vi "4 Axis - Set Absolute Target Position.vi"(4 "error in (no error)":errorcluster, 5 "Positions":sgl[](array[numeric]), 7 "Controller Reference In":refnum<k7>) -> (0 "error out":errorcluster, 3 "Controller Reference Out":refnum<k7>)   [LabVIEW 2015]
doc: "Sets all 4 axis target positions (Absolute positions)."
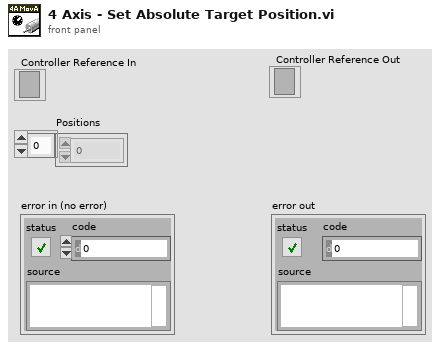
[diagram p1: front panel]
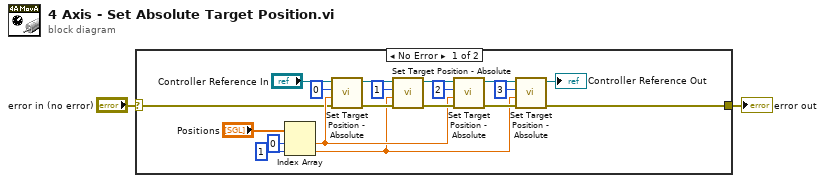
[diagram p0: block diagram]
diagram:
  n1 = case shown="No Error" "error in (no error)" {
    selector: "error in (no error)" -> [w3 w22]
    tunnel: [w4 w22] -> w2
    frame No Error {
      n2 = Index Array(array="Positions", index #1=0 ("index"), index #2=1 ("index")) -> (element #1=w8:sgl, element #2=w7:sgl)
      n3 = call "Set Target Position - Absolute.vi"("error in (no error)"=w3, "Target Position"=w8, "Axis In"=i16 0, "Controller Reference In"="Controller Reference In") -> ("error out"=w18:errorcluster, "Controller Reference Out"=w19:refnum<k7>)  [unwired: 1 in, 1 out]
      n4 = call "Set Target Position - Absolute.vi"("error in (no error)"=w18, "Target Position"=w7, "Axis In"=i16 1, "Controller Reference In"=w19) -> ("error out"=w16:errorcluster, "Controller Reference Out"=w17:refnum<k7>)  [unwired: 1 in, 1 out]
      n5 = call "Set Target Position - Absolute.vi"("error in (no error)"=w16, "Target Position"=w8, "Axis In"=i16 2, "Controller Reference In"=w17) -> ("error out"=w14:errorcluster, "Controller Reference Out"=w15:refnum<k7>)  [unwired: 1 in, 1 out]
      n6 = call "Set Target Position - Absolute.vi"("error in (no error)"=w14, "Target Position"=w7, "Axis In"=i16 3, "Controller Reference In"=w15) -> ("error out"=w4:errorcluster, "Controller Reference Out"=→"Controller Reference Out":refnum<k7>)  [unwired: 1 in, 1 out]
    }
    frame Error {
    }
  }
  "error out" <- w2
